vi "Get Run Number.vi"(11 "AnytimeDStar in":refnum<class "NI_Robotics_AnytimeDStar.lvclass">) -> (2 "run number":i32, 3 "AnytimeDStar out":refnum<class "NI_Robotics_AnytimeDStar.lvclass">)   [LabVIEW 2017, in "NI_Robotics_AnytimeDStar.lvclass"]
uses:
  <vilib>/robotics/Navigation/Anytime D Star/NI_Robotics_AnytimeDStar.lvclass
  <vilib>/robotics/Navigation/Anytime D Star/NI_Robotics_AnytimeDStar.lvclass/NI_Robotics_AnytimeDStar.ctl
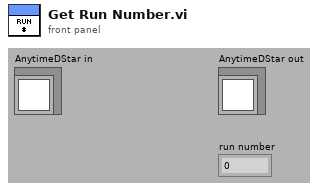
[diagram p1: front panel]
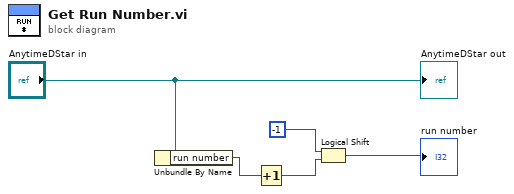
[diagram p0: block diagram]
diagram:
  n1 = Unbundle By Name("AnytimeDStar in") -> ("run number"=w3:i32)
  n2 = Increment(x=w3) -> (x+1=w2:i32)
  n3 = Logical Shift(y=-1 ("x"), x=w2) -> (x << y=→"run number":i32)
  "AnytimeDStar out" <- "AnytimeDStar in"
